vi "step.vi"(1 "n":i32=1, 2 "v":dbl=10.0, 3 "z":dbl, 4 "y":dbl, 5 "x":dbl, 6 "连接ID":refnum<k5>) -> (0 "连接ID":refnum<k5>)   [LabVIEW 2017]
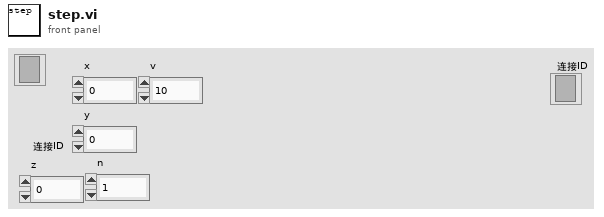
[diagram p1: front panel]
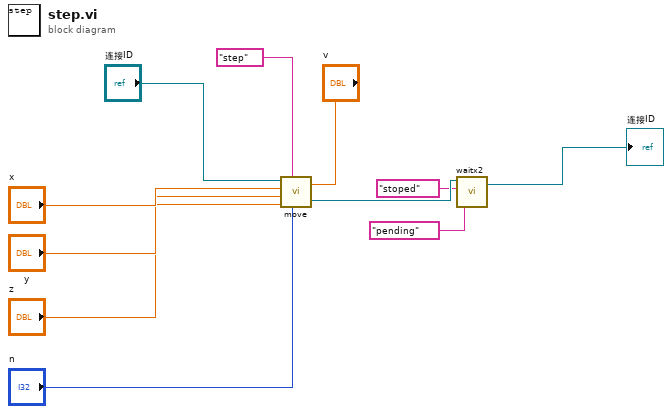
[diagram p0: block diagram]
diagram:
  n1 = call "move.vi"("v"="v", "n"="n", "String"="step", "z"="z", "y"="y", "x"="x", "连接ID"="连接ID") -> ("连接ID输出"=w4:refnum<k5>)
  n2 = call "waitx2.vi"("String Value 2"="pending", "String Value"="stoped", "连接ID"=w4) -> ("连接ID 2"=→"连接ID":refnum<k5>)  [unwired: 1 in, 1 out]
